vi "Projectile.vi"() -> ()   [LabVIEW 2015]
uses:
  <vilib>/imath/engines/lvmath2/RunTimeEngine/Managers/WorkSpace/UID Generator.vi
  <vilib>/imath/engines/lvmath2/RunTimeEngine/RunTimeType/NIMS_RunTimeType_From StrictType (excl LVString).vi
  <instcachedir>/0/NIMS_RunTimeType_From StrictType (excl LVString)_EB1C38A9BC5048DA9ABDA8F781E54D21.lvgen/NIMS_RunTimeType_From StrictType (excl LVString)_EB1C38A9BC5048DA9ABDA8F781E54D21_000.vi
  <vilib>/imath/engines/lvmath2/RunTimeEngine/LocalVariableDefStatement/MC_LocalVariableDefStatement_Display.vi
  <vilib>/imath/engines/lvmath2/RunTimeEngine/Managers/SymbolTable/Clear UID.vi
  <vilib>/imath/engines/lvmath2/RunTimeEngine/NodeEndStatement/NIMS_NodeEndStatement_Output.vi
  <instcachedir>/0/NIMS_NodeEndStatement_Output_53EC0D466D134D7ABD903AC30B43404B.lvgen/NIMS_NodeEndStatement_Output_53EC0D466D134D7ABD903AC30B43404B_009.vi
  <vilib>/imath/engines/lvmath2/RunTimeEngine/ErrorHandling/NIMS_Finalize Error.vi
  <vilib>/imath/engines/lvmath2/RunTimeEngine/Managers/SymbolTable/NIMS_WorkSpace.lvlib
panel:
  out "XY Graph":cluster{i32[], dbl[]}(graph)
  in  "Launch Height (m)":dbl
  in  "Launch Speed (m/s)":dbl
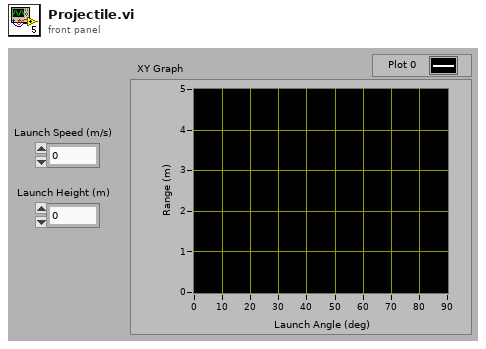
[diagram p1: front panel]
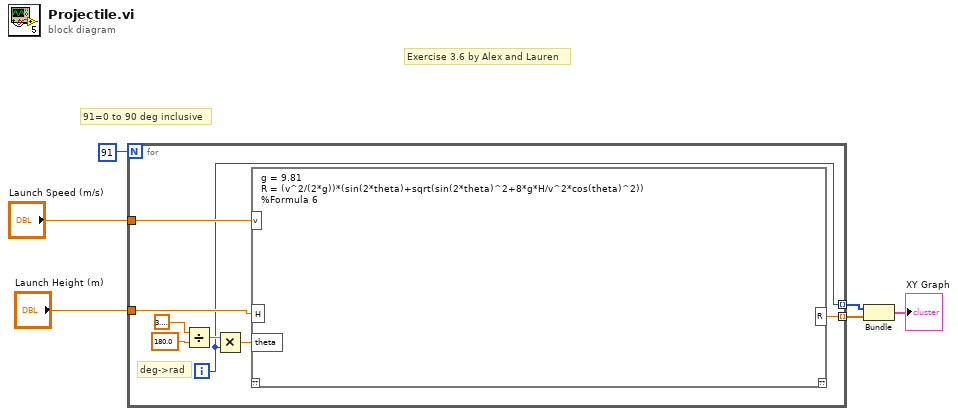
[diagram p0: block diagram]
diagram:
  # "91=0 to 90 deg inclusive"
  # "Exercise 3.6 by Alex and Lauren"
  n1 = for {
    N: 91 -> [_]
    tunnel: [w7] -> w6 mode=indexing
    tunnel: "Launch Speed (m/s)" -> [w14]
    tunnel: "Launch Height (m)" -> [w13]
    tunnel: [w8] -> w2 mode=indexing
    i -> [w8]
    # "deg->rad"
    n2 = Divide(x=3.141592653589793, y=180.0) -> (x/y=w10:dbl)
    n3 = Multiply(x=w10, y=w8) -> (x*y=w9:dbl)
    n4 = mathscript code="g = 9.81\nR = (v^2/(2*g))*(sin(2*theta)+sqrt(sin(2*theta)^2+8*g*H/v^2*cos(theta)^2))\n%Formula 6"("v"=w14, "H"=w13, "theta"=w9) -> ("R"=w7:cdb)  [unwired: 1 in, 1 out]
  }
  n5 = Bundle(w2, w6) -> (→"XY Graph":cluster{i32[], cdb[]})  [unwired: 1 in]
